vi "Proximity.vi"(0 "data":string) -> (1 "distance":dbl, 2 "proximity":bool, 3 "max":dbl)   [LabVIEW 2014]
doc: "Extracts the proximity information from the sensor-data"
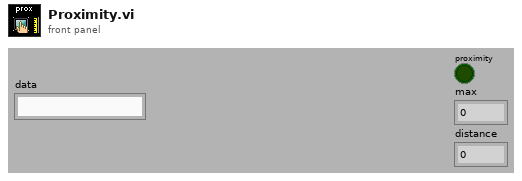
[diagram p1: front panel]
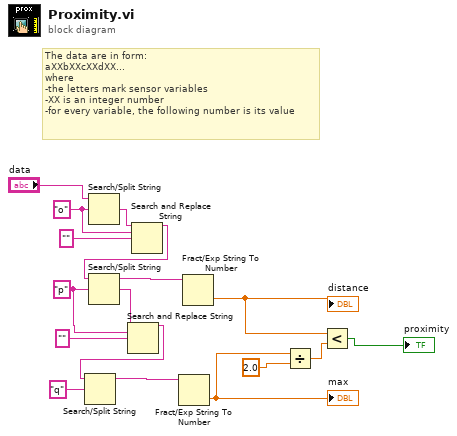
[diagram p0: block diagram]
diagram:
  w6 = "p" ("search string/char (-)")
  w16 = "o" ("search string/char (-)")
  # "The data are in form:\naXXbXXcXXdXX...\nwhere \n-the letters mark sensor variables\n-XX is an integer number\n-for every variable, the following number is its value"
  n1 = Search/Split String(string="data", search string/char (-)=w16) -> (match + rest of string=w15:string)  [unwired: 1 in, 2 out]
  n2 = Search and Replace String(input string=w15, search string=w16, replace string="" ("replace string (\"\")")) -> (result string=w14:string)  [unwired: 5 in, 3 out]
  n3 = Search/Split String(string=w14, search string/char (-)=w6) -> (substring before match=w13:string, match + rest of string=w8:string)  [unwired: 1 in, 1 out]
  n4 = Search and Replace String(input string=w8, search string=w6, replace string="" ("replace string (\"\")")) -> (result string=w7:string)  [unwired: 5 in, 3 out]
  n5 = Search/Split String(string=w7, search string/char (-)="q") -> (substring before match=w9:string)  [unwired: 1 in, 2 out]
  n6 = Fract/Exp String To Number(string=w9) -> (number=w3:dbl)  [unwired: 3 in, 1 out]
  "max" <- w3
  n7 = Fract/Exp String To Number(string=w13) -> (number=w5:dbl)  [unwired: 3 in, 1 out]
  "distance" <- w5
  n8 = Divide(x=w3, y=2.0) -> (x/y=w2:dbl)
  n9 = Less?(x=w5, y=w2) -> (x < y?=→"proximity":bool)
